vi "Run Test - Log Condition (SubVI).vi"(8 "error in (no error)":errorcluster, 10 "Time":dbl, 11 "Cluster in":T1 {"M Event" items=["Stop", "Running", "PID", "Up Limit", "Down Limit", "Load Limit"]; "Test Type" items=["Please Select", "Triaxial Shear", "Triaxial UU", "Shearbox", "Permeability", "Consolidation (Stepped Loading)/Swelling", "Saturation (Incremental)", "User Defined", "UCT", "Isotropic Consolidation", "Swelling Pressure"]; "Data"."Test Type" items=["Please Select", "Triaxial Shear", "Triaxial UU", "Shearbox", "Permeability", "Consolidation (Stepped Loading)/Swelling", "Saturation (Incremental)", "User Defined", "UCT", "Isotropic Consolidation", "Swelling Pressure"]}) -> (0 "error out":errorcluster, 3 "Cluster out":T1 {"M Event" items=["Stop", "Running", "PID", "Up Limit", "Down Limit", "Load Limit"]; "Test Type" items=["Please Select", "Triaxial Shear", "Triaxial UU", "Shearbox", "Permeability", "Consolidation (Stepped Loading)/Swelling", "Saturation (Incremental)", "User Defined", "UCT", "Isotropic Consolidation", "Swelling Pressure"]; "Data"."Test Type" items=["Please Select", "Triaxial Shear", "Triaxial UU", "Shearbox", "Permeability", "Consolidation (Stepped Loading)/Swelling", "Saturation (Incremental)", "User Defined", "UCT", "Isotropic Consolidation", "Swelling Pressure"]}, 5 "Enum":T10)   [LabVIEW 2019]
uses:
  Controls/RunTest - State.ctl
  Controls/RunTest - Data Structure.ctl
  Controls/Test Panel - Data Structure.ctl
  Controls/Station - Test Type.ctl
  <vilib>/Utility/miscctls.llb/LVRowAndColumnTypeDef.ctl
  Controls/RunTest - Calculate Data.ctl
  <vilib>/httpClient/ClientHandle.ctl
  Controls/RunTest - Start Condition.ctl
  Controls/RunTest - Stop Condition.ctl
  Controls/UDP - Event.ctl
  <vilib>/httpClient/LabVIEWHTTPClient.lvlib
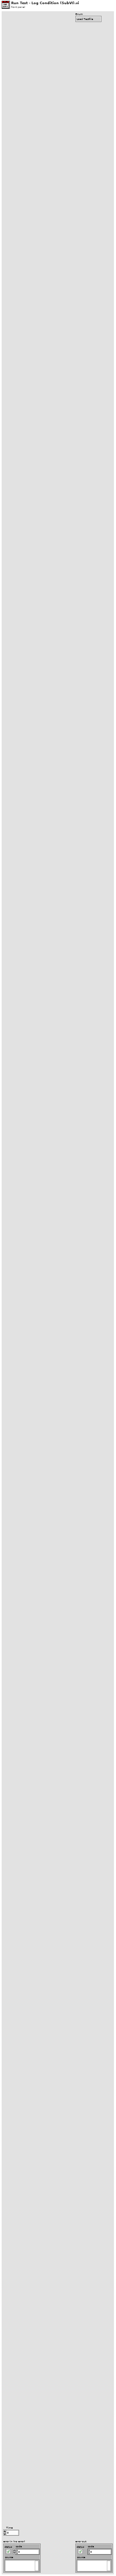
[diagram p1: front panel]
types:
  T1 = typedef "RunTest - Data Structure.ctl" = cluster{"Test Plan":string[], "PlanRow":i32, "Device Name":string[], "Timeout":i32, "Start?":bool, "Pause?":bool, "IP Address":string[], "LogRow":i32, "Logtype":u16, "Log Elapse":sgl, "Data":T2, "Stop log?":bool, "tdms":refnum<k34>, "Sensor Data":sgl[], "Start time":timestamp, "Prev Log Elapse":u32, "Plot":u16, "X-Axis":u16[], "Y-Axis":u16[], "XY":cluster{"X":dbl, "Y":dbl}[][], "End Stage?":bool, "1run":bool, "Condition":u16[], "Start Con":bool, "Log Con":bool, "Stop Con":bool, "Start Elapse":dbl, "Start Load":dbl, "Motor":i32, "StartRow":i32, "number log":i32, "Dir":bool, "Start time test":timestamp, "Auto":bool, "Check return?":bool, "Inv":cluster{"M":i32[], "Bool":bool[]}, "tdms temp":refnum<k34>, "Zero?":bool, "Plot Timer":dbl, "1st Run":bool, "TDMS Path":path, "MaxLoad":dbl, "Log Timer":sgl[], "Test Type":T3, "Log Sensor":string[], "Save?":bool, "1st Log":bool, "Y-Axis 2":u16[], "On Y-Axis 2":bool, "Decimal":u8[], "Init":cluster{"PWP TS":sgl, "Load TS":sgl, "Volume TS":sgl, "Disp TS":sgl, "CP":sgl, "Vol In":sgl, "Vol Out":sgl, "Load UCT":sgl, "Disp UCT":sgl, "PWP Sat":sgl, "CP Sat":sgl, "Volume IsoCons":sgl, "PWP IsoCons":sgl, "PWP TUU":sgl, "Load TUU":sgl, "Volume TUU":sgl, "Disp TUU":sgl, "Load Cons":sgl, "Disp Cons":sgl, "Volume Sat":sgl, "Vertical Load SB":sgl, "Vertical Disp SB":sgl, "H Disp SB":sgl, "H Load SB":sgl}, "Calc":T5, "Device Index":i32[], "Channel Index":i32[], "http ref":T6, "fileid":string, "Step Cons":cluster{"V Stress":sgl, "H Settlement":sgl}, "RunTest":bool, "Graph Last":i32, "Init?":bool, "Datalog":bool[], "Start":T7, "Stop":T8, "Running?":bool, "StartTime":dbl, "Log Prev Time":dbl, "KeyName":string[], "Test RunTime":dbl, "Log Prev Axial":dbl, "M Event":T9[], "Last Log":bool, "popup":bool, "PreStart UU":bool, "PreStart Sat":bool}
  T2 = typedef "Test Panel - Data Structure.ctl" = cluster{"Station":string, "Sample ID":string, "Job No":string, "Job Description":string, "Filename":string, "Test Type":T3, "Speciment No":string, "Depth":string, "Height":string, "Diameter/Length":string, "Weight":string, "Test Parameter":string, "Station[]":string[], "Edit Pos":T4, "Edit Pos Prev":T4, "Area":string, "Path":string}
  T3 = typedef "Station - Test Type.ctl" = u16
  T4 = typedef "LVRowAndColumnTypeDef.ctl" = cluster{"Row":i32, "Column":i32}
  T5 = typedef "RunTest - Calculate Data.ctl" = cluster{"TS":cluster{"Change PWP":sgl, "Change Vol":sgl, "Axial Load":sgl, "CiL":sgl, "Deviator":sgl, "Axial Strain":sgl, "MaxDeviator":sgl}, "TUU":cluster{"Change PWP":sgl, "Axial Load":sgl, "CiL":sgl, "Deviator":sgl, "Axial Strain":sgl, "MaxDeviator":sgl}, "Sat":cluster{"B Value":sgl, "PWP Diss":sgl, "CPP":sgl, "CV":sgl}, "Per":cluster{"Change Vol In":sgl, "Change Vol Out":sgl, "Mean Vol":sgl, "Gradient Pressure":sgl, "Outlet Flow":sgl, "Inlet Flow":sgl, "I X1":sgl, "I X2":sgl, "I Y1":sgl, "I Y2":sgl, "O X1":sgl, "O X2":sgl, "O Y1":sgl, "O Y2":sgl}, "Step Cons":cluster{"V Stress":sgl, "H Settlement":sgl, "Total H Settle":sgl, "Prev Total H":sgl}, "UCT":cluster{"ALC":sgl, "H Change":sgl, "Deviator":sgl, "Axial Strain":sgl, "V Stress":sgl, "MaxDeviator":sgl}, "ISO Cons":cluster{"CPP":sgl, "PWP Diss":sgl, "CV":sgl}, "SB":cluster{"Speci LenC":sgl, "Shear Strain":sgl, "H LC":sgl, "Normal Stress":sgl, "Shear Stress":sgl, "MaxShear":sgl}}
  T6 = typedef "LabVIEWHTTPClient.lvlib/ClientHandle.ctl" = refnum<k1>
  T7 = typedef "RunTest - Start Condition.ctl" = cluster{"Cons":cluster{"VS":dbl, "Delay":bool, "No Delay":dbl}, "Sat":cluster{"CP":dbl, "BP":dbl, "StartBP":bool, "Target CP":bool, "Target BP":bool}, "Iso":cluster{"Select":dbl, "BP":dbl, "IC2":dbl, "IC3":dbl, "IC4":dbl, ". IC6":bool, "IC6":dbl, "IC6-2":dbl, "Target":bool, "Time Cond":dbl, "Last PWP":dbl}, "TS":cluster{"SS":dbl, "Engage":bool, "ES":dbl, "LC":dbl, "PreStart":bool, "Trig SS":bool, "Drain":dbl}, "TUU":cluster{"SS":dbl, "Engage":bool, "ES":dbl, "LC":dbl, "PreStart":bool, "Trig SS":bool, "CP":dbl, "Delay Value":dbl, "Delay":bool, "CP PID":bool}, "UCT":cluster{"SS":dbl, "Engage":bool, "ES":dbl, "LC":dbl, "PreStart":bool, "Trig SS":bool}, "Enable?":bool, "SB":cluster{"SS":dbl, "Engage":bool, "ES":dbl, "LC":dbl, "PreStart":bool, "Trig SS":bool, "VS":dbl, "Delay Value":dbl, "Delay":bool, "VS PID":bool}, "Perm":cluster{"DP":dbl}}
  T8 = typedef "RunTest - Stop Condition.ctl" = cluster{"Cons":cluster{"Select":i32, "Disp":dbl, "Time":dbl, "Time2":dbl, "Disp 2":dbl, "Time Cond":dbl, "Last Disp":dbl, "Swell":bool}, "Sat":cluster{"Select":i32, "PP":dbl, "Time":dbl, "VC":dbl, "Time2":dbl, "Time Cond":dbl, "Last PP":dbl, ".B":bool, "B":dbl, "Last Vc":dbl, "Time Cond 2":dbl, "Time3":dbl, "Time Cond 3":dbl, "B Achieve":bool}, "Iso":cluster{"PP":dbl, "Time":dbl, "VC":dbl, "Time2":dbl, "Time Cond":dbl, "Last Vc":dbl, ".PP":bool, "Time Cond 2":dbl, "Select":i32}, "TS":cluster{"Axial":dbl, ".MaxDev":bool, "MaxDev Value":dbl, "Return":bool, "Reset":bool, "Prev Time":dbl, "PostStop Run":bool, "CP Stop":bool, "BP Stop":bool, "PostStop Trig":bool, "Reset Value":dbl, "BPTrig":bool, "CPTrig":bool, "VLCTrig":bool}, "TUU":cluster{"Axial":dbl, ".MaxDev":bool, "MaxDev Value":dbl, "Return":bool, "Reset":bool, "Prev Time":dbl, "PostStop Run":bool, "CP Stop":bool, "BP Stop":bool, "PostStop Trig":bool, "Reset Value":dbl, "BPTrig":bool, "CPTrig":bool, "VLCTrig":bool}, "UCT":cluster{"Axial":dbl, ".MaxDev":bool, "MaxDev Value":dbl, "Return":bool, "Reset":bool, "Prev Time":dbl, "PostStop Run":bool, "CP Stop":bool, "BP Stop":bool, "PostStop Trig":bool}, "Enable?":bool, "SB":cluster{"Shear":dbl, ".MaxShear":bool, "MaxShear Value":dbl, "Return":bool, "Reset":bool, "Prev Time":dbl, "PostStop Run":bool, "CP Stop":bool, "BP Stop":bool, "PostStop Trig":bool, "Reset Value":dbl, "BPTrig":bool, "CPTrig":bool, "VLCTrig":bool}, "Perm":cluster{"Max Time":bool, "Reset":bool, "PostStop Run":bool, "Ratio":bool, "Reset Value":dbl, "Time":dbl, "RatioTime":dbl, "RatioMore":dbl, "RatioLess":dbl, "Time Cond":dbl, "Time Cond 2":dbl, "Prev IF":dbl, "Prev OF":dbl, "PostStop Trig":bool, "BP Trig":bool, "DP Stop":bool, "BP Stop":bool, "CP Stop":bool, "CP Trig":bool}, "SP":cluster{".Max Time":bool, ".Time":bool, "Time":dbl, "MaxTime":dbl, "Time Cond":dbl, "Max Time Cond":dbl, "Stress":dbl}}
  T9 = typedef "UDP - Event.ctl" = u16
  T10 = typedef "RunTest - State.ctl" = enum16{"Load Testfile", "Notifier", "Init", "Idle", "Load", "Read DB", "Run", "Pause", "Stop", "Check Start", "Check Stop", "Check Post Stop", "Check Log", "EndStage", "Data View", "Display", "Graph", "Graph Old", "Close", "Stop PID", "Check Limit", "Auto", "Up", "Log", "Zero", "Machine Control", "Save Report"}
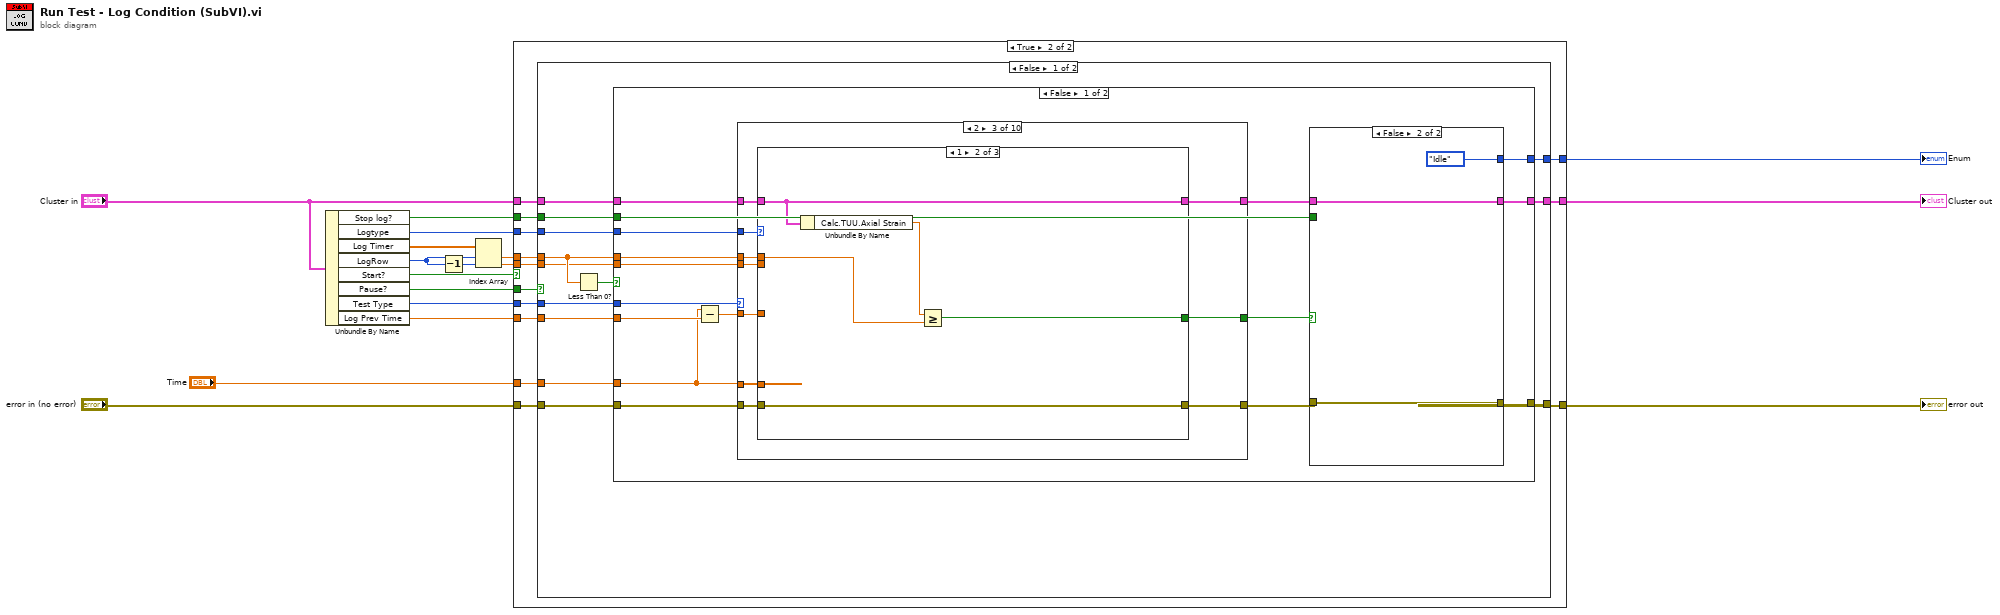
[diagram p0: block diagram]
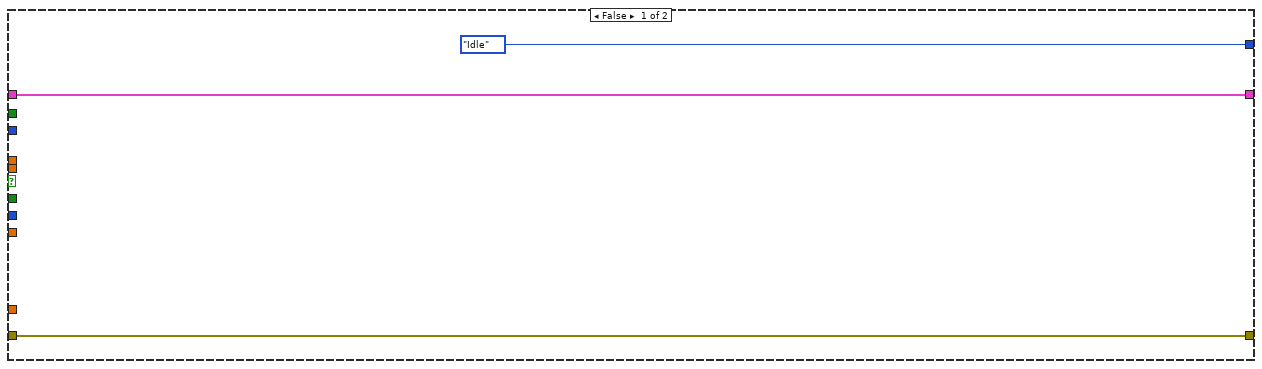
[diagram p2: hidden frame]
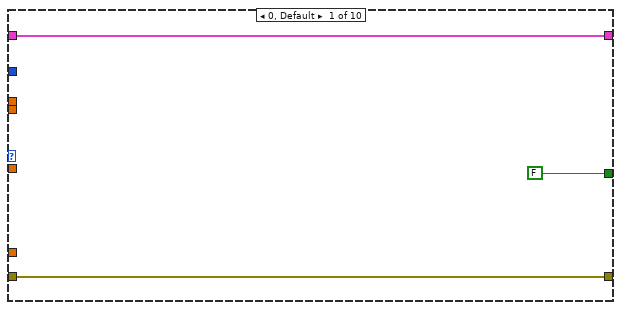
[diagram p3: hidden frame]
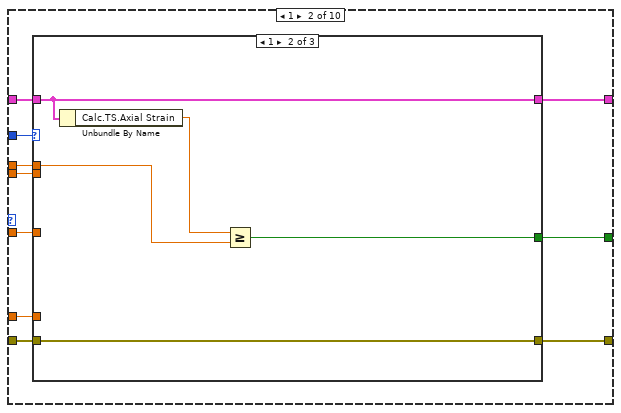
[diagram p4: hidden frame]
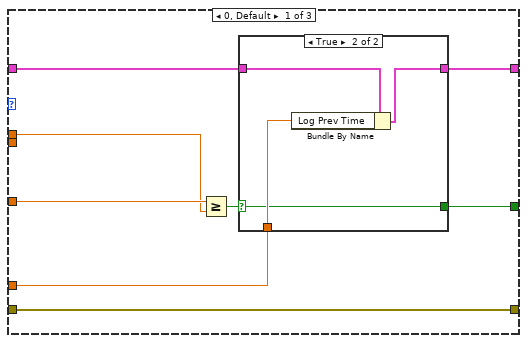
[diagram p5: hidden frame]
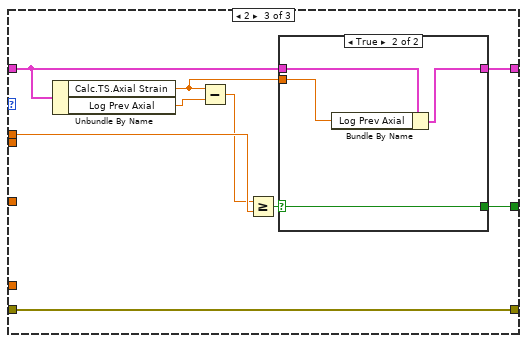
[diagram p7: hidden frame]
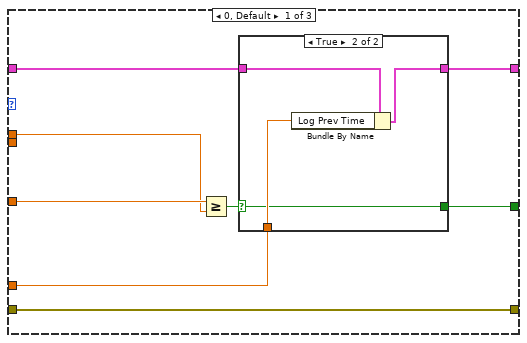
[diagram p9: hidden frame]
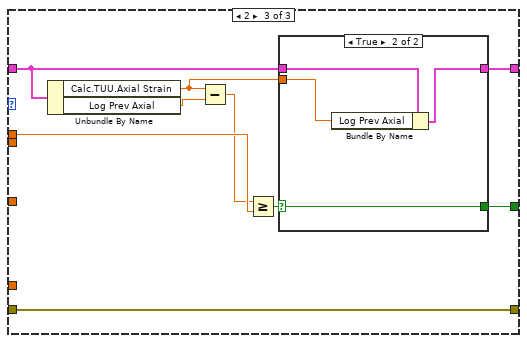
[diagram p11: hidden frame]
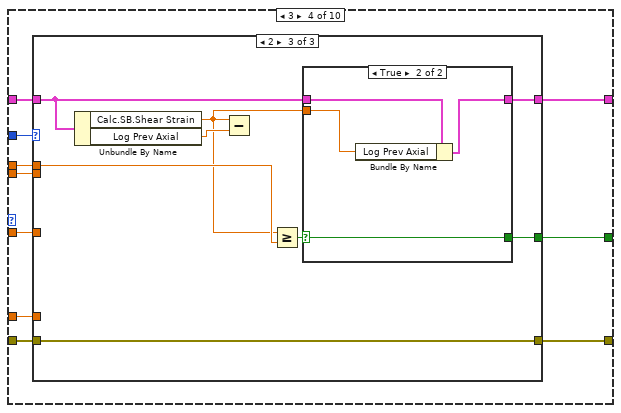
[diagram p13: hidden frame]
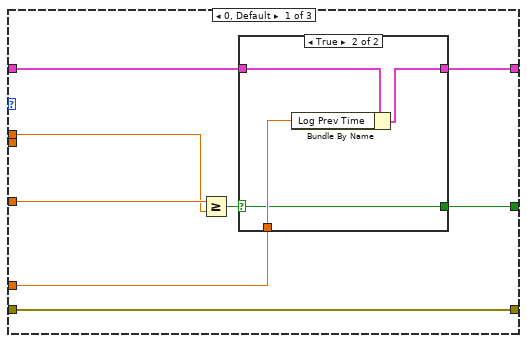
[diagram p14: hidden frame]
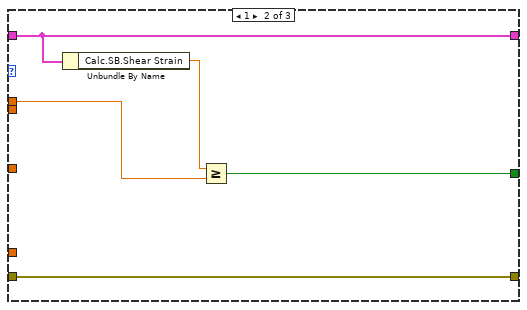
[diagram p16: hidden frame]
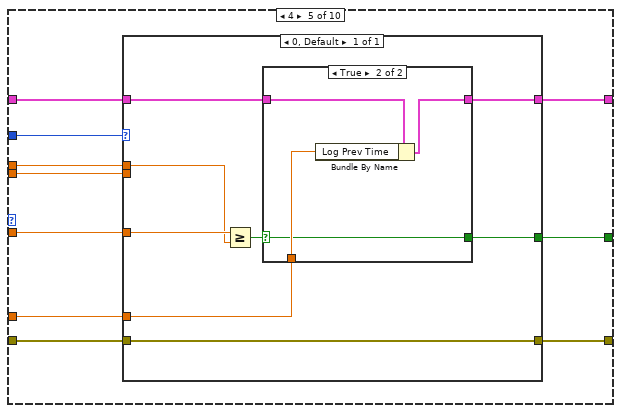
[diagram p18: hidden frame]
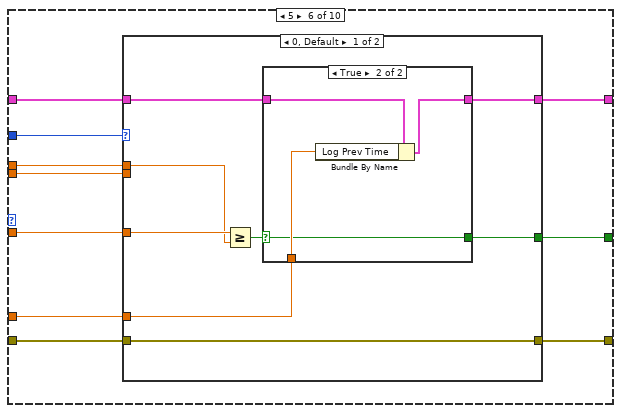
[diagram p20: hidden frame]
diagram:
  n1 = Unbundle By Name("Cluster in") -> ("Stop log?"=w11:bool, "Logtype"=w10:u16, "Log Timer"=w8:sgl[], "LogRow"=w14:i32, "Start?"=w1:bool, "Pause?"=w2:bool, "Test Type"=w12:T3, "Log Prev Time"=w16:dbl)
  n2 = Decrement(x=w14) -> (x-1=w13:i32)
  n3 = Index Array(array=w8, index #1=w14, index #2=w13) -> (element #1=w9:sgl, element #2=w15:sgl)
  n4 = case shown="True" w1 {
    tunnel: [RunTest_-_State."Idle" w33] -> w7
    tunnel: "error in (no error)" -> [w19 w32]
    tunnel: [w20 w31] -> w5
    tunnel: "Cluster in" -> [w20 w30]
    tunnel: [w19 w29] -> w6
    tunnel: w9 -> [_ w28]
    tunnel: w2 -> [_ w27]
    tunnel: w10 -> [_ w26]
    tunnel: w11 -> [_ w25]
    tunnel: w12 -> [_ w24]
    tunnel: w15 -> [_ w23]
    tunnel: w16 -> [_ w22]
    tunnel: "Time" -> [_ w21]
    frame False {
    }
    frame True {
      n5 = case shown="False" w27 {
        tunnel: [w46 RunTest_-_State."Idle"] -> w33
        tunnel: w32 -> [w45 w422]
        tunnel: [w44 w423] -> w31
        tunnel: w30 -> [w43 w423]
        tunnel: [w42 w422] -> w29
        tunnel: w28 -> [w41 _]
        tunnel: w26 -> [w39 _]
        tunnel: w25 -> [w38 _]
        tunnel: w24 -> [w37 _]
        tunnel: w23 -> [w36 _]
        tunnel: w22 -> [w35 _]
        tunnel: w21 -> [w34 _]
        frame False {
          n6 = Less Than 0?(x=w41) -> (x < 0?=w40:bool)
          n7 = case shown="False" w40 {
            tunnel: [w62 RunTest_-_State."Display"] -> w46
            tunnel: w45 -> [w49 w419]
            tunnel: [w61 w420] -> w44
            tunnel: w43 -> [w50 w420]
            tunnel: [w60 w419] -> w42
            tunnel: w41 -> [w58 _]
            tunnel: w39 -> [w57 _]
            tunnel: w38 -> [w56 _]
            tunnel: w37 -> [w55 _]
            tunnel: w36 -> [w54 _]
            tunnel: w35 -> [w53 _]
            tunnel: w34 -> [w48 _]
            frame False {
              n8 = Subtract(x=w48, y=w53) -> (x-y=w52:dbl)
              n9 = case shown="2" w55 {
                tunnel: w52 -> [_ w75 w119 w163 w206 w230 w270 w310 w354 w394]
                tunnel: w58 -> [_ w74 w118 w162 w205 w229 w269 w309 w353 w393]
                tunnel: [w65 w73 w117 w161 w204 w228 w268 w308 w352 w392] -> w51
                tunnel: w50 -> [w65 w72 w116 w160 w203 w227 w267 w307 w351 w391]
                tunnel: w48 -> [_ w71 w115 w159 w202 w226 w266 w306 w350 w390]
                tunnel: [FALSE w70 w114 w158 w201 w225 w265 w305 w349 w389] -> w47
                tunnel: [w63 w69 w113 w157 w200 w224 w264 w304 w348 w388] -> w59
                tunnel: w49 -> [w63 w68 w112 w156 w199 w223 w263 w303 w347 w387]
                tunnel: w57 -> [_ w67 w111 w155 w198 w222 w262 w302 w346 w386]
                tunnel: w54 -> [_ w66 w110 w154 w197 w221 w261 w301 w345 w385]
                frame 0, Default {
                }
                frame 1 {
                  n10 = case shown="1" w67 {
                    tunnel: w75 -> [w83 _ _]
                    tunnel: w74 -> [w82 w90 w103]
                    tunnel: [w81 w92 w102] -> w73
                    tunnel: w72 -> [w80 w92 w98]
                    tunnel: w71 -> [w79 _ _]
                    tunnel: [w77 w94 w100] -> w70
                    tunnel: [w76 w93 w99] -> w69
                    tunnel: w68 -> [w76 w93 w99]
                    tunnel: w66 -> [_ _ _]
                    frame 0, Default {
                      n11 = Greater Or Equal?(x=w83, y=w82) -> (x >= y?=w78:bool)
                      n12 = case shown="True" w78 {
                        selector: w78 -> [w84 w86]
                        tunnel: [w85 w89] -> w81
                        tunnel: w80 -> [w85 w88]
                        tunnel: w79 -> [_ w87]
                        tunnel: [w84 w86] -> w77
                        frame False {
                        }
                        frame True {
                          n13 = Bundle By Name(cluster=w88, "Log Prev Time"=w87) -> (w89:T1)
                        }
                      }
                    }
                    frame 1 {
                      n14 = Unbundle By Name(w92) -> ("Calc.TS.Axial Strain"=w91:sgl)
                      n15 = Greater Or Equal?(x=w91, y=w90) -> (x >= y?=w94:bool)
                    }
                    frame 2 {
                      n16 = Unbundle By Name(w98) -> ("Calc.TS.Axial Strain"=w95:sgl, "Log Prev Axial"=w97:dbl)
                      n17 = Subtract(x=w95, y=w97) -> (x-y=w96:dbl)
                      n18 = Greater Or Equal?(x=w96, y=w103) -> (x >= y?=w101:bool)
                      n19 = case shown="True" w101 {
                        selector: w101 -> [w104 w107]
                        tunnel: [w105 w109] -> w102
                        tunnel: w98 -> [w105 w108]
                        tunnel: [w104 w107] -> w100
                        tunnel: w95 -> [_ w106]
                        frame False {
                        }
                        frame True {
                          n20 = Bundle By Name(cluster=w108, "Log Prev Axial"=w106) -> (w109:T1)
                        }
                      }
                    }
                  }
                }
                frame 2 {
                  n21 = case shown="1" w111 {
                    tunnel: w119 -> [w127 _ _]
                    tunnel: w118 -> [w126 w134 w147]
                    tunnel: [w125 w136 w146] -> w117
                    tunnel: w116 -> [w124 w136 w142]
                    tunnel: w115 -> [w123 _ _]
                    tunnel: [w121 w138 w144] -> w114
                    tunnel: [w120 w137 w143] -> w113
                    tunnel: w112 -> [w120 w137 w143]
                    tunnel: w110 -> [_ _ _]
                    frame 0, Default {
                      n22 = Greater Or Equal?(x=w127, y=w126) -> (x >= y?=w122:bool)
                      n23 = case shown="True" w122 {
                        selector: w122 -> [w128 w130]
                        tunnel: [w129 w133] -> w125
                        tunnel: w124 -> [w129 w132]
                        tunnel: w123 -> [_ w131]
                        tunnel: [w128 w130] -> w121
                        frame False {
                        }
                        frame True {
                          n24 = Bundle By Name(cluster=w132, "Log Prev Time"=w131) -> (w133:T1)
                        }
                      }
                    }
                    frame 1 {
                      n25 = Unbundle By Name(w136) -> ("Calc.TUU.Axial Strain"=w135:sgl)
                      n26 = Greater Or Equal?(x=w135, y=w134) -> (x >= y?=w138:bool)
                    }
                    frame 2 {
                      n27 = Unbundle By Name(w142) -> ("Calc.TUU.Axial Strain"=w140:sgl, "Log Prev Axial"=w141:dbl)
                      n28 = Subtract(x=w140, y=w141) -> (x-y=w139:dbl)
                      n29 = Greater Or Equal?(x=w139, y=w147) -> (x >= y?=w145:bool)
                      n30 = case shown="True" w145 {
                        selector: w145 -> [w148 w151]
                        tunnel: [w149 w153] -> w146
                        tunnel: w142 -> [w149 w152]
                        tunnel: [w148 w151] -> w144
                        tunnel: w140 -> [_ w150]
                        frame False {
                        }
                        frame True {
                          n31 = Bundle By Name(cluster=w152, "Log Prev Axial"=w150) -> (w153:T1)
                        }
                      }
                    }
                  }
                }
                frame 3 {
                  n32 = case shown="2" w155 {
                    tunnel: w163 -> [w171 _ _]
                    tunnel: w162 -> [w170 w178 w190]
                    tunnel: [w169 w180 w189] -> w161
                    tunnel: w160 -> [w168 w180 w185]
                    tunnel: w159 -> [w167 _ _]
                    tunnel: [w165 w182 w187] -> w158
                    tunnel: [w164 w181 w186] -> w157
                    tunnel: w156 -> [w164 w181 w186]
                    tunnel: w154 -> [_ _ _]
                    frame 0, Default {
                      n33 = Greater Or Equal?(x=w171, y=w170) -> (x >= y?=w166:bool)
                      n34 = case shown="True" w166 {
                        selector: w166 -> [w172 w174]
                        tunnel: [w173 w177] -> w169
                        tunnel: w168 -> [w173 w176]
                        tunnel: w167 -> [_ w175]
                        tunnel: [w172 w174] -> w165
                        frame False {
                        }
                        frame True {
                          n35 = Bundle By Name(cluster=w176, "Log Prev Time"=w175) -> (w177:T1)
                        }
                      }
                    }
                    frame 1 {
                      n36 = Unbundle By Name(w180) -> ("Calc.SB.Shear Strain"=w179:sgl)
                      n37 = Greater Or Equal?(x=w179, y=w178) -> (x >= y?=w182:bool)
                    }
                    frame 2 {
                      n38 = Unbundle By Name(w185) -> ("Calc.SB.Shear Strain"=w183:sgl, "Log Prev Axial"=w184:dbl)
                      n39 = Subtract(x=w183, y=w184) -> ()  [unwired: 1 out]
                      n40 = Greater Or Equal?(x=w183, y=w190) -> (x >= y?=w188:bool)
                      n41 = case shown="True" w188 {
                        selector: w188 -> [w191 w194]
                        tunnel: [w192 w196] -> w189
                        tunnel: w185 -> [w192 w195]
                        tunnel: [w191 w194] -> w187
                        tunnel: w183 -> [_ w193]
                        frame False {
                        }
                        frame True {
                          n42 = Bundle By Name(cluster=w195, "Log Prev Axial"=w193) -> (w196:T1)
                        }
                      }
                    }
                  }
                }
                frame 4 {
                  n43 = case shown="0, Default" w198 {
                    tunnel: w206 -> [w214]
                    tunnel: w205 -> [w213]
                    tunnel: [w212] -> w204
                    tunnel: w203 -> [w211]
                    tunnel: w202 -> [w210]
                    tunnel: [w208] -> w201
                    tunnel: [w207] -> w200
                    tunnel: w199 -> [w207]
                    tunnel: w197 -> [_]
                    frame 0, Default {
                      n44 = Greater Or Equal?(x=w214, y=w213) -> (x >= y?=w209:bool)
                      n45 = case shown="True" w209 {
                        selector: w209 -> [w215 w217]
                        tunnel: [w216 w220] -> w212
                        tunnel: w211 -> [w216 w219]
                        tunnel: w210 -> [_ w218]
                        tunnel: [w215 w217] -> w208
                        frame False {
                        }
                        frame True {
                          n46 = Bundle By Name(cluster=w219, "Log Prev Time"=w218) -> (w220:T1)
                        }
                      }
                    }
                  }
                }
                frame 5 {
                  n47 = case shown="0, Default" w222 {
                    tunnel: w230 -> [w238 w254]
                    tunnel: w229 -> [w237 w245]
                    tunnel: [w236 w253] -> w228
                    tunnel: w227 -> [w235 w252]
                    tunnel: w226 -> [w234 w251]
                    tunnel: [w232 w249] -> w225
                    tunnel: [w231 w248] -> w224
                    tunnel: w223 -> [w231 w248]
                    tunnel: w221 -> [_ w247]
                    frame 0, Default {
                      n48 = Greater Or Equal?(x=w238, y=w237) -> (x >= y?=w233:bool)
                      n49 = case shown="True" w233 {
                        selector: w233 -> [w239 w241]
                        tunnel: [w240 w244] -> w236
                        tunnel: w235 -> [w240 w243]
                        tunnel: w234 -> [_ w242]
                        tunnel: [w239 w241] -> w232
                        frame False {
                        }
                        frame True {
                          n50 = Bundle By Name(cluster=w243, "Log Prev Time"=w242) -> (w244:T1)
                        }
                      }
                    }
                    frame 1 {
                      n51 = Subtract(x=w245, y=w247) -> (x-y=w246:sgl)
                      n52 = Greater Or Equal?(x=w254, y=w246) -> (x >= y?=w250:bool)
                      n53 = case shown="True" w250 {
                        selector: w250 -> [w255 w257]
                        tunnel: [w256 w260] -> w253
                        tunnel: w252 -> [w256 w259]
                        tunnel: w251 -> [_ w258]
                        tunnel: [w255 w257] -> w249
                        frame False {
                        }
                        frame True {
                          n54 = Bundle By Name(cluster=w259, "Log Prev Time"=w258) -> (w260:T1)
                        }
                      }
                    }
                  }
                }
                frame 6 {
                  # "Saturation"
                  n55 = case shown="1" w262 {
                    tunnel: w270 -> [w278 w294]
                    tunnel: w269 -> [w277 w285]
                    tunnel: [w276 w293] -> w268
                    tunnel: w267 -> [w275 w292]
                    tunnel: w266 -> [w274 w291]
                    tunnel: [w272 w289] -> w265
                    tunnel: [w271 w288] -> w264
                    tunnel: w263 -> [w271 w288]
                    tunnel: w261 -> [_ w287]
                    frame 0, Default {
                      n56 = Greater Or Equal?(x=w278, y=w277) -> (x >= y?=w273:bool)
                      n57 = case shown="True" w273 {
                        selector: w273 -> [w279 w281]
                        tunnel: [w280 w284] -> w276
                        tunnel: w275 -> [w280 w283]
                        tunnel: w274 -> [_ w282]
                        tunnel: [w279 w281] -> w272
                        frame False {
                        }
                        frame True {
                          n58 = Bundle By Name(cluster=w283, "Log Prev Time"=w282) -> (w284:T1)
                        }
                      }
                    }
                    frame 1 {
                      n59 = Subtract(x=w285, y=w287) -> (x-y=w286:sgl)
                      n60 = Greater Or Equal?(x=w294, y=w286) -> (x >= y?=w290:bool)
                      n61 = case shown="True" w290 {
                        selector: w290 -> [w295 w297]
                        tunnel: [w296 w300] -> w293
                        tunnel: w292 -> [w296 w299]
                        tunnel: w291 -> [_ w298]
                        tunnel: [w295 w297] -> w289
                        frame False {
                        }
                        frame True {
                          n62 = Bundle By Name(cluster=w299, "Log Prev Time"=w298) -> (w300:T1)
                        }
                      }
                    }
                  }
                }
                frame 8 {
                  n63 = case shown="1" w302 {
                    tunnel: w310 -> [w318 _ _]
                    tunnel: w309 -> [w317 w325 w338]
                    tunnel: [w316 w327 w337] -> w308
                    tunnel: w307 -> [w315 w327 w333]
                    tunnel: w306 -> [w314 _ _]
                    tunnel: [w312 w329 w335] -> w305
                    tunnel: [w311 w328 w334] -> w304
                    tunnel: w303 -> [w311 w328 w334]
                    tunnel: w301 -> [_ _ _]
                    frame 0, Default {
                      n64 = Greater Or Equal?(x=w318, y=w317) -> (x >= y?=w313:bool)
                      n65 = case shown="True" w313 {
                        selector: w313 -> [w319 w321]
                        tunnel: [w320 w324] -> w316
                        tunnel: w315 -> [w320 w323]
                        tunnel: w314 -> [_ w322]
                        tunnel: [w319 w321] -> w312
                        frame False {
                        }
                        frame True {
                          n66 = Bundle By Name(cluster=w323, "Log Prev Time"=w322) -> (w324:T1)
                        }
                      }
                    }
                    frame 1 {
                      n67 = Unbundle By Name(w327) -> ("Calc.UCT.Axial Strain"=w326:sgl)
                      n68 = Greater Or Equal?(x=w326, y=w325) -> (x >= y?=w329:bool)
                    }
                    frame 2 {
                      n69 = Unbundle By Name(w333) -> ("Calc.UCT.Axial Strain"=w330:sgl, "Log Prev Axial"=w332:dbl)
                      n70 = Subtract(x=w330, y=w332) -> (x-y=w331:dbl)
                      n71 = Greater Or Equal?(x=w331, y=w338) -> (x >= y?=w336:bool)
                      n72 = case shown="True" w336 {
                        selector: w336 -> [w339 w342]
                        tunnel: [w340 w344] -> w337
                        tunnel: w333 -> [w340 w343]
                        tunnel: [w339 w342] -> w335
                        tunnel: w330 -> [_ w341]
                        frame False {
                        }
                        frame True {
                          n73 = Bundle By Name(cluster=w343, "Log Prev Axial"=w341) -> (w344:T1)
                        }
                      }
                    }
                  }
                }
                frame 9 {
                  n74 = case shown="0, Default" w346 {
                    tunnel: w354 -> [w362 w378]
                    tunnel: w353 -> [w361 w369]
                    tunnel: [w360 w377] -> w352
                    tunnel: w351 -> [w359 w376]
                    tunnel: w350 -> [w358 w375]
                    tunnel: [w356 w373] -> w349
                    tunnel: [w355 w372] -> w348
                    tunnel: w347 -> [w355 w372]
                    tunnel: w345 -> [_ w371]
                    frame 0, Default {
                      n75 = Greater Or Equal?(x=w362, y=w361) -> (x >= y?=w357:bool)
                      n76 = case shown="True" w357 {
                        selector: w357 -> [w363 w365]
                        tunnel: [w364 w368] -> w360
                        tunnel: w359 -> [w364 w367]
                        tunnel: w358 -> [_ w366]
                        tunnel: [w363 w365] -> w356
                        frame False {
                        }
                        frame True {
                          n77 = Bundle By Name(cluster=w367, "Log Prev Time"=w366) -> (w368:T1)
                        }
                      }
                    }
                    frame 1 {
                      n78 = Subtract(x=w369, y=w371) -> (x-y=w370:sgl)
                      n79 = Greater Or Equal?(x=w378, y=w370) -> (x >= y?=w374:bool)
                      n80 = case shown="True" w374 {
                        selector: w374 -> [w379 w381]
                        tunnel: [w380 w384] -> w377
                        tunnel: w376 -> [w380 w383]
                        tunnel: w375 -> [_ w382]
                        tunnel: [w379 w381] -> w373
                        frame False {
                        }
                        frame True {
                          n81 = Bundle By Name(cluster=w383, "Log Prev Time"=w382) -> (w384:T1)
                        }
                      }
                    }
                  }
                }
                frame 10 {
                  n82 = case shown="0, Default" w386 {
                    tunnel: w394 -> [w402]
                    tunnel: w393 -> [w401]
                    tunnel: [w400] -> w392
                    tunnel: w391 -> [w399]
                    tunnel: w390 -> [w398]
                    tunnel: [w396] -> w389
                    tunnel: [w395] -> w388
                    tunnel: w387 -> [w395]
                    tunnel: w385 -> [_]
                    frame 0, Default {
                      n83 = Greater Or Equal?(x=w402, y=w401) -> (x >= y?=w397:bool)
                      n84 = case shown="True" w397 {
                        selector: w397 -> [w403 w405]
                        tunnel: [w404 w408] -> w400
                        tunnel: w399 -> [w404 w407]
                        tunnel: w398 -> [_ w406]
                        tunnel: [w403 w405] -> w396
                        frame False {
                        }
                        frame True {
                          n85 = Bundle By Name(cluster=w407, "Log Prev Time"=w406) -> (w408:T1)
                        }
                      }
                    }
                  }
                }
              }
              n86 = case shown="False" w47 {
                tunnel: [w411 RunTest_-_State."Idle"] -> w62
                tunnel: [w413 w416] -> w61
                tunnel: w51 -> [w413 w416]
                tunnel: [w414 w417] -> w60
                tunnel: w59 -> [w414 w417]
                tunnel: w56 -> [w412 _]
                frame True {
                  n87 = Select(t=RunTest_-_State."Idle", s=w412, f=RunTest_-_State."Log") -> (s? t:f=w411:T10)
                }
                frame False {
                }
              }
            }
            frame True {
            }
          }
        }
        frame True {
        }
      }
    }
  }
  "Enum" <- w7
  "error out" <- w6
  "Cluster out" <- w5
